vi "ViewLine.vi"(7 "Header format":u16(ring) items=["Riverside Format", "Ron Linear"], 10 "Line #":i32, 11 "new file path":path=path "C:/WINDOWS/DESKTOP/rri.eye") -> (2 "sample rate MHz":u16, 3 "Waveform Graph":i16[](graph))   [LabVIEW 2022 SP3]
panel:
  out "# lines per scan":u16
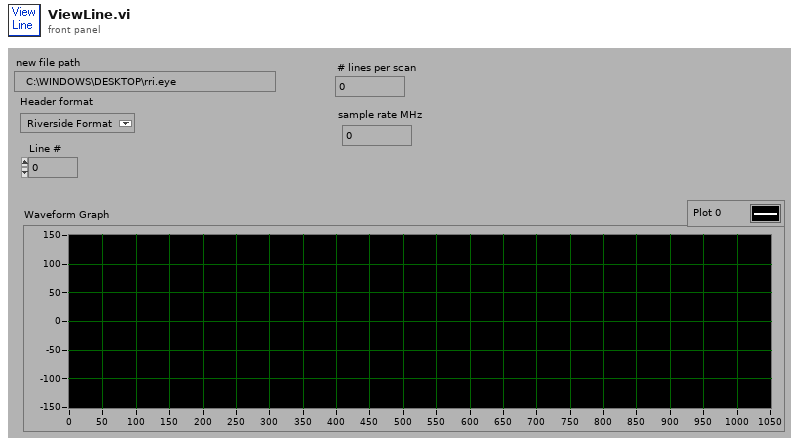
[diagram p1: front panel]
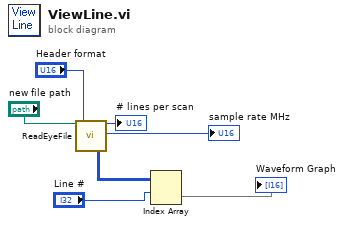
[diagram p0: block diagram]
diagram:
  n1 = call "ReadEyeFile.vi"("new file path"="new file path", "Header format"="Header format") -> ("2-D data array"=w5:i16[][], "# lines per scan"=→"# lines per scan":u16, "sample rate MHz"=→"sample rate MHz":u16)  [unwired: 15 out]
  n2 = Index Array(array=w5, index (row)="Line #") -> (element=→"Waveform Graph":i16[])  [unwired: 1 in]
